vi "Set Up Daq.vi"(8 "Use Ephys":bool, 10 "Number of samples per s":dbl, 11 "Array":waveform(dbl)[](array[waveform])) -> (2 "task out 2":refnum<k21>, 3 "Refnum out":refnum<k21>)   [LabVIEW 2018]
uses:
  <vilib>/DAQmx/write.llb/DAQmx Write (Analog 1D Wfm NChan NSamp).vi
  <vilib>/DAQmx/create/channels.llb/DAQmx Create Channel (AO-Voltage-Basic).vi
  <vilib>/DAQmx/configure/timing.llb/DAQmx Timing (Sample Clock).vi
  <vilib>/DAQmx/miscellaneous.llb/DAQmx Fill In Error Info.vi
  <vilib>/DAQmx/create/channels.llb/DAQmx Create Channel (AI-Voltage-Basic).vi
  <resource>/objmgr/daqmx.rc
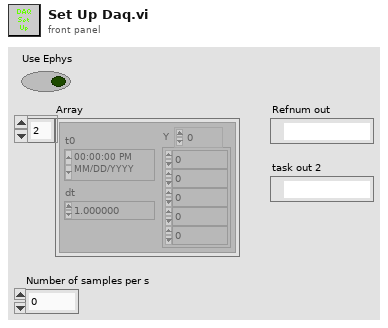
[diagram p1: front panel]
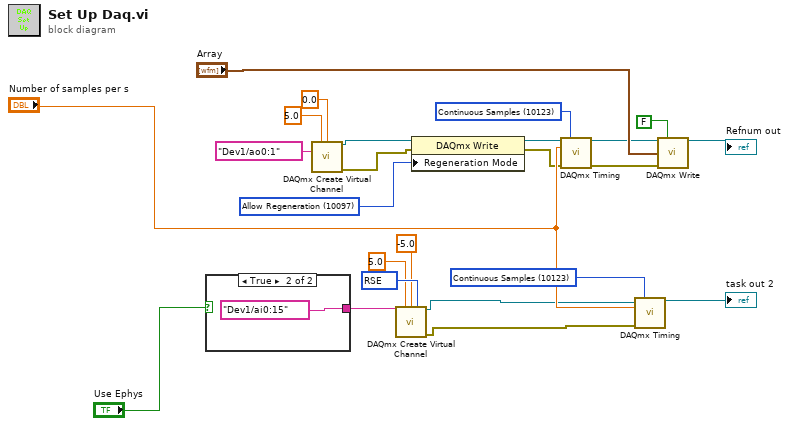
[diagram p0: block diagram]
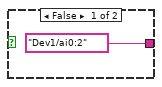
[diagram p2: hidden frame]
diagram:
  w14 = 10083 items=["Default"=-1, "RSE"=10083, "NRSE"=10078, "Differential"=10106, "Pseudodifferential"=12529] ("input terminal configuration")
  w13 = 10123 items=["Finite Samples"=10178, "Continuous Samples"=10123, "Hardware Timed Single Point"=12522] ("sample mode")
  w11 = 10123 items=["Finite Samples"=10178, "Continuous Samples"=10123, "Hardware Timed Single Point"=12522] ("sample mode")
  w5 = 10097 items=["Allow Regeneration"=10097, "Do Not Allow Regeneration"=10158] ("RegenMode")
  n1 = case shown="True" "Use Ephys" {
    tunnel: [tag "Dev1/ai0:2" ("physical channels") tag "Dev1/ai0:15" ("physical channels")] -> w12
    frame False {
    }
    frame True {
    }
  }
  n2 = call-poly <vilib>:"DAQmx Create Virtual Channel.vi"("maximum value"=5.0, "minimum value"=0.0, "physical channels"=tag "Dev1/ao0:1") -> ("task out"=w4:refnum<k21>, "error out"=w8:errorcluster)  [unwired: 11 in]
  n3 = call-poly <vilib>:"DAQmx Create Virtual Channel.vi"("maximum value"=5.0, "minimum value"=-5.0, "input terminal configuration"=w14, "physical channels"=w12) -> ("task out"=w21:refnum<k21>, "error out"=w22:errorcluster)  [unwired: 10 in]
  n4 = property class="DAQmx Write"(reference=w4, error in=w8, "Regeneration Mode"=w5) -> (reference out=w10:refnum<k21>, error out=w9:errorcluster)
  n5 = call-poly <vilib>:"DAQmx Timing.vi"("task/channels in"=w10, "sample mode"=w11, "rate"="Number of samples per s", "error in"=w9) -> ("task out"=w18:refnum<k21>, "error out"=w20:errorcluster)  [unwired: 10 in]
  n6 = call-poly <vilib>:"DAQmx Timing.vi"("task/channels in"=w21, "sample mode"=w13, "rate"="Number of samples per s", "error in"=w22) -> ("task out"=→"task out 2":refnum<k21>)  [unwired: 10 in, 1 out]
  n7 = call-poly <vilib>:"DAQmx Write.vi"("task/channels in"=w18, "auto start"=FALSE, "data"="Array", "error in"=w20) -> ("task out"=→"Refnum out":refnum<k21>)  [unwired: 9 in, 2 out]
